vi "AutoExtracOpt-simulation.vi"() -> ()   [LabVIEW 2020]
uses:
  subvi/status/StopSoftware.vi
  subvi/status/Tip_No_300.vi
  subvi/status/Tip_No_1000.vi
  subvi/status/Vial_No.vi
  subvi/status/Liquid_List.vi
  subvi/status/Log.vi
  subvi/status/LogCSVName.vi
  subvi/status/ExtracOptOperations.vi
  subvi/status/ExtracOptDeviceStatus.vi
  subvi/status/ExtracOptTaskStatus.vi
  subvi/status/ExtracOptConversationId.vi
  subvi/status/ExtracOptTaskId.vi
  subvi/status/EmergencyStop.vi
  subvi/status/ExtracOptCommand.vi
panel:
  out "ExtracOptConversationId":string
  out "ExtracOptTaskId":string
  out "ExtracOptDeviceStatus":string
  out "ExtracOptOperations":string
  out "Current_1000 uL_Tip_No":i32
  out "Current_300 uL_Tip_No":i32
  out "Current_Vial_No":i32
  out "Current_Log":string
  in  "Device_Log":i32(listbox)=-1
  in  "StopSoftware":bool
  in  "Control":enum32{"Auto", "Manual", "system"}(tab)
  in  "Data_Record":bool
  in  "Change_Vial&Tip_No":bool
  in  "Vial_No":i32
  in  "Tip_No_1000":i32
  in  "Tip_No_300":i32
  out "Array":string[][](array[string])
  out "ExtracOptCommand":string
  in  "EmergencyStop":bool
  # "1-10"
  # "89"
  # "1"
  # "4"
  # "2"
  # "→"
  # "→"
  # "1"
  # "3"
  # "8"
  # "96"
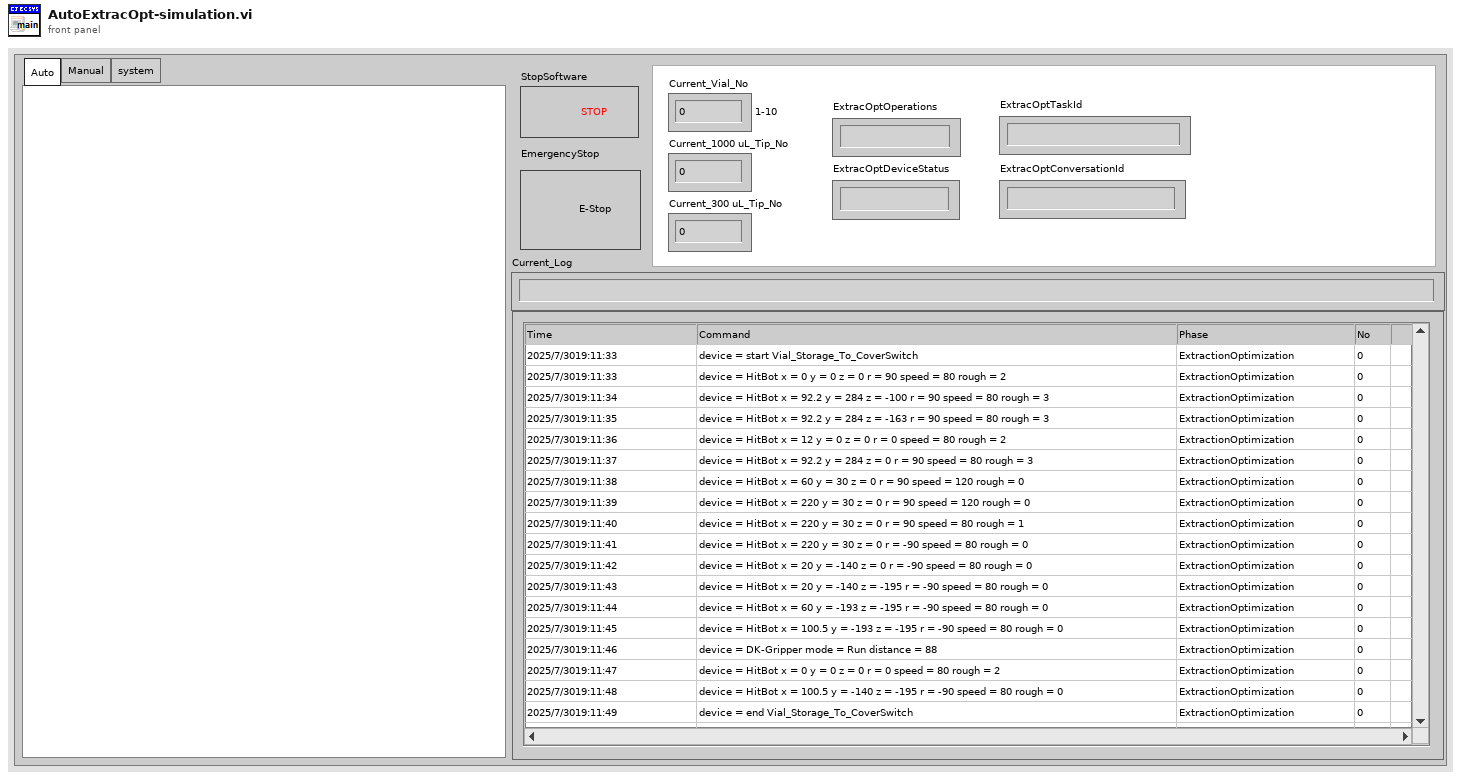
[diagram p1: front panel]
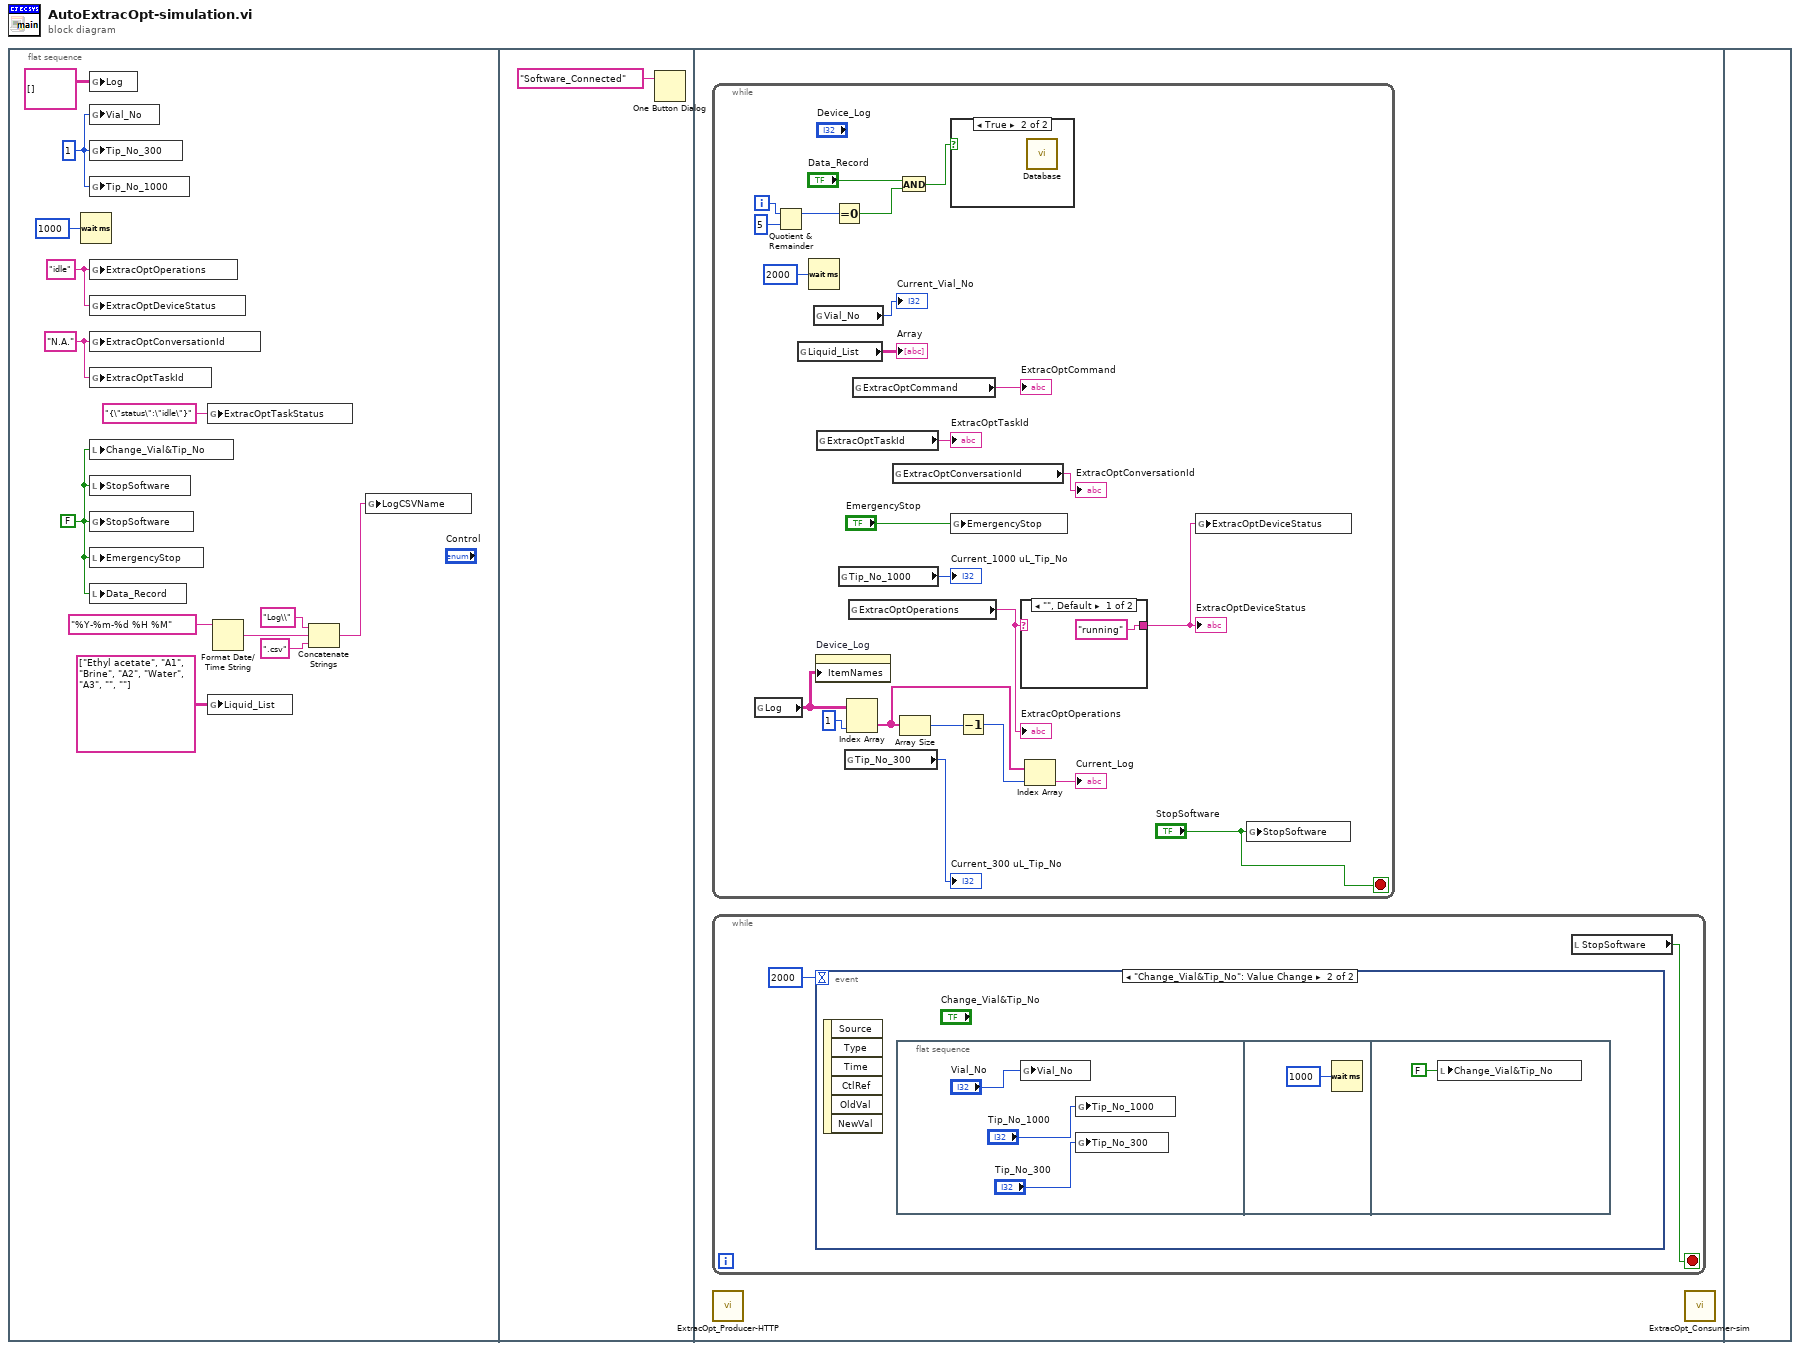
[diagram p0: block diagram]
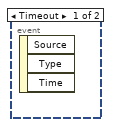
[diagram p2: hidden frame]
diagram:
  n1 = flat-sequence {
    frame #0 {
      w2 = "N.A." ("ReactorTemp")
      w4 = "idle" ("Operations")
      w11 = 1 ("Vial_No")
      w1 = FALSE ("stop software")
      n2 = Wait (ms)(milliseconds to wait=u32 1000) -> ()  [unwired: 1 out]
      n3 = global write "Log.vi" "Log"(string[][] [] ("Log")) -> ()
      n4 = global write "Vial_No.vi" "Vial_No"(w11) -> ()
      n5 = global write "Tip_No_300.vi" "Tip_No_300"(w11) -> ()
      n6 = global write "Tip_No_1000.vi" "Tip_No_1000"(w11) -> ()
      n7 = global write "ExtracOptOperations.vi" "ExtracOptOperations"(w4) -> ()
      n8 = global write "ExtracOptDeviceStatus.vi" "ExtracOptDeviceStatus"(w4) -> ()
      n9 = global write "ExtracOptConversationId.vi" "ExtracOptConversationId"(w2) -> ()
      n10 = global write "ExtracOptTaskId.vi" "ExtracOptTaskId"(w2) -> ()
      n11 = local write "Change_Vial&Tip_No"(w1) -> ()
      n12 = local write "StopSoftware"(w1) -> ()
      n13 = global write "StopSoftware.vi" "StopSoftware"(w1) -> ()
      n14 = local write "EmergencyStop"(w1) -> ()
      n15 = local write "Data_Record"(w1) -> ()
      n16 = global write "ExtracOptTaskStatus.vi" "ExtracOptTaskStatus"("{\"status\":\"idle\"}" ("ReactionImagePath")) -> ()
      n17 = global write "Liquid_List.vi" "Liquid_List"(string[][] [["Ethyl acetate", "A1"], ["Brine", "A2"], ["Water", "A3"], ["", ""]] ("Liquid_List")) -> ()
      n18 = Format Date/Time String(time format string (%c)="%Y-%m-%d %H %M") -> (date/time string=w10:string)  [unwired: 2 in]
      n19 = Concatenate Strings("Log\\" ("string"), w10, ".csv" ("string")) -> (w9:string)
      n20 = global write "LogCSVName.vi" "LogCSVName"(w9) -> ()
    }
    frame #1 {
      n21 = One Button Dialog(message="Software_Connected") -> ()  [unwired: 1 in, 1 out]
    }
    frame #2 {
      n22 = while {
        i -> [w27]
        stop <- "StopSoftware" stop-if-true
        n23 = global read "Log.vi" "Log"() -> (w34:string[][])
        n24 = Quotient & Remainder(x=w27, y=5) -> (x-y*floor(x/y)=w25:i32)  [unwired: 1 out]
        n25 = global read "Liquid_List.vi" "Liquid_List"() -> (→"Array":string[][])
        n26 = Wait (ms)(milliseconds to wait=u32 2000) -> ()  [unwired: 1 out]
        n27 = global read "Vial_No.vi" "Vial_No"() -> (→"Current_Vial_No":i32)
        n28 = property on="Device_Log" class="MCListbox (strict)"("ItemNames"=w34) -> ()  [unwired: 2 in, 2 out]
        n29 = global read "ExtracOptTaskId.vi" "ExtracOptTaskId"() -> (→"ExtracOptTaskId":string)
        n30 = Equal To 0?(x=w25) -> (x = 0?=w23:bool)
        n31 = global read "Tip_No_1000.vi" "Tip_No_1000"() -> (→"Current_1000 uL_Tip_No":i32)
        n32 = global read "Tip_No_300.vi" "Tip_No_300"() -> (→"Current_300 uL_Tip_No":i32)
        n33 = Index Array(array=w34, index (col)=1 ("index (row)")) -> (element=w39:string[])  [unwired: 1 in]
        n34 = global read "ExtracOptOperations.vi" "ExtracOptOperations"() -> (w32:string)
        "ExtracOptOperations" <- w32
        n35 = global read "ExtracOptCommand.vi" "ExtracOptCommand"() -> (→"ExtracOptCommand":string)
        n36 = global read "ExtracOptConversationId.vi" "ExtracOptConversationId"() -> (→"ExtracOptConversationId":string)
        n37 = And(x="Data_Record", y=w23) -> (x .and. y?=w22:bool)
        n38 = Array Size(array=w39) -> (size(s)=w36:i32)
        n39 = case shown="True" w22 {
          frame False {
          }
          frame True {
            n40 = call "Database.vi"() -> ()  [unwired: 11 in, 1 out]
          }
        }
        n41 = global write "EmergencyStop.vi" "EmergencyStop"("EmergencyStop") -> ()
        n42 = Decrement(x=w36) -> (x-1=w35:i32)
        n43 = case shown="\"\", Default" w32 {
          selector: w32 -> [_ w47]
          tunnel: ["running" ("ReactionDeviceStatus") w47] -> w31
          frame "", Default {
          }
          frame "idle" {
          }
        }
        "ExtracOptDeviceStatus" <- w31
        n44 = Index Array(array=w39, index=w35) -> (element=→"Current_Log":string)
        n45 = global write "ExtracOptDeviceStatus.vi" "ExtracOptDeviceStatus"(w31) -> ()
        n46 = global write "StopSoftware.vi" "StopSoftware"("StopSoftware") -> ()
      }
      n47 = while {
        stop <- w16 stop-if-true
        n48 = event shown="[1] \"Change_Vial&Tip_No\": Value Change" {
          selector: _ -> [_ _]
          dyn-events: _ -> [_ _]
          timeout: 2000 -> [_ _]
          event Timeout {
            n49 = event-data() -> ()  [unwired: 1 in, 3 out]
          }
          event "Change_Vial&Tip_No": Value Change {
            n50 = event-data() -> ()  [unwired: 1 in, 6 out]
            n51 = flat-sequence {
              frame #0 {
                n52 = global write "Vial_No.vi" "Vial_No"("Vial_No") -> ()
                n53 = global write "Tip_No_1000.vi" "Tip_No_1000"("Tip_No_1000") -> ()
                n54 = global write "Tip_No_300.vi" "Tip_No_300"("Tip_No_300") -> ()
              }
              frame #1 {
                n55 = Wait (ms)(milliseconds to wait=u32 1000) -> ()  [unwired: 1 out]
              }
              frame #2 {
                n56 = local write "Change_Vial&Tip_No"(FALSE ("Add_Vial_No")) -> ()
              }
            }
          }
        }
        n57 = local read "StopSoftware"() -> (w16:bool)
      }
      n58 = call "ExtracOpt_Producer-HTTP.vi"() -> ()  [unwired: 12 in]
      n59 = call "ExtracOpt_Consumer-sim.vi"() -> ()  [unwired: 12 in]
    }
    frame #3 {
    }
  }
